vi "NISE.Execute Command.vi"   [LabVIEW 2016, in "SLSC Interface.lvclass"]
uses:
  SLSC Interface.lvclass
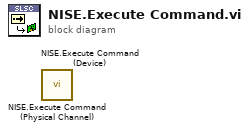
[diagram p0: block diagram]
diagram:
  n1 = call "NISE.Execute Command (Physical Channel).vi"() -> ()  [unwired: 14 in, 2 out]
  n2 = call "NISE.Execute Command (Device).vi"() -> ()  [unwired: 14 in, 2 out]
